vi "test Work Directory.vi"(8 "error in":errorcluster) -> (0 "error out":errorcluster)   [LabVIEW 2024, in "serenial.io-ase.test.lvlib"]
uses:
  serenial.io-ase.test.lvlib
  <vilib>/addons/_JKI Toolkits/Caraya/classes/Test/Test.lvclass
  serenial.io-ase/ase/ase.lvclass
  <vilib>/addons/_JKI Toolkits/Caraya/classes/Assert/Assert.lvclass
  <vilib>/addons/_JKI Toolkits/Caraya/classes/Assert/Assert Equal Value_Variant.vi
  serenial.io-ase/ase/Start Call (Command).vi
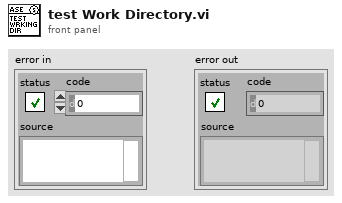
[diagram p1: front panel]
types:
  T1 = typedef "serenial.io-ase.lvlib/ase.lvclass/Event References.ctl" = cluster{"Standard Output":refnum<user-event>, "Standard Error":refnum<user-event>, "Did Exit":refnum<user-event>}
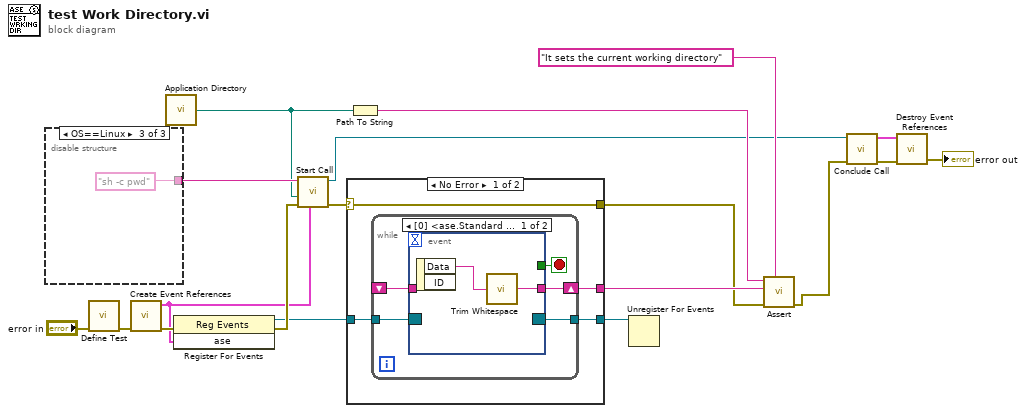
[diagram p0: block diagram]
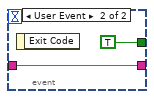
[diagram p2: hidden frame]
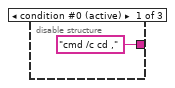
[diagram p4: hidden frame]
diagram:
  n1 = disable-structure "Conditional Disable Structure" shown="OS==Linux" {
    disable-tunnel: ["cmd /c cd ," _ "sh -c pwd"] -> w9
    frame condition #0 (active) {
    }
    frame condition #1 {
    }
    frame condition #2 {
    }
  }
  n2 = call <vilib>:"Define Test.vi"("error in (no error)"="error in") -> ("error out"=w17:errorcluster)  [unwired: 9 in, 1 out]
  n3 = call "Create Event References.vi"("error in"=w17) -> ("error out"=w18:errorcluster, "ase"=w6:T1)  [unwired: 9 in]
  n4 = call <vilib>:"Application Directory.vi"() -> ("Application Directory"=w8:path)
  n5 = register-events(error in=w18, w6) -> (reference out=w14:refnum<event-registration>, error out=w16:errorcluster)  [unwired: 1 in]
  n6 = call-poly "Start Call.vi"("Event References"=w6, "error in"=w16, "Working Directory (default <Not A Path> - System Default)"=w8, "Command"=w9) -> ("error out"=w15:errorcluster, "New ASE Handle"=w5:refnum<class "ase.lvclass">)  [unwired: 6 in]
  n7 = case shown="No Error" w15 {
    selector: w15 -> [w25 w36]
    tunnel: w14 -> [w24 w35]
    tunnel: [w23 _] -> w11
    tunnel: [w22 w35] -> w13
    tunnel: [w25 w36] -> w7
    frame No Error {
      n8 = while {
        tunnel: w24 -> [w30]
        tunnel: [w28] -> w22
        shift-right: [w27] -> w23
        shift-left: _ -> [w26]
        stop <- w29 stop-if-true
        n9 = event shown="[0] <ase.Standard Output>: User Event" {
          selector: w30 -> [_ _]
          dyn-events: [_ _] -> w28
          timeout: _ -> [_ _]
          tunnel: [_ TRUE] -> w29
          tunnel: [w31 w33] -> w27
          tunnel: w26 -> [_ w33]
          event User Event {
            n10 = event-data() -> ("Data"=w32:string)  [unwired: 1 in, 1 out]
            n11 = call <vilib>:"Trim Whitespace.vi"("string"=w32) -> ("trimmed string"=w31:string)  [unwired: 1 in]
          }
          event User Event {
            n12 = event-data() -> ()  [unwired: 1 in, 1 out]
          }
        }
      }
    }
    frame Error {
    }
  }
  n13 = Path To String(path=w8) -> (string=w12:string)
  n14 = Unregister For Events(event registration refnum=w13) -> ()  [unwired: 1 in, 1 out]
  n15 = call-poly <vilib>:"Assert.vi"("Label"="It sets the current working directory", "error in (no error)"=w7, "Y"=w11, "X"=w12) -> ("error out"=w4:errorcluster)  [unwired: 6 in, 1 out]
  n16 = call "Conclude Call.vi"("error in"=w4, "ASE Handle"=w5) -> ("error out"=w3:errorcluster, "Event References"=w1:T1)  [unwired: 7 in, 1 out]
  n17 = call "Destroy Event References.vi"("error in"=w3, "Event References"=w1) -> ("error out"=→"error out":errorcluster)  [unwired: 9 in]
